vi "Example_Multiple.vi"() -> ()   [LabVIEW 2015, in "LXM32_Modbus_Serial.lvlib"]
uses:
  LXM32_Modbus_Serial.lvlib
  register_param.ctl
  <vilib>/Utility/sysdir.llb/System Directory Type.ctl
  <vilib>/Utility/file.llb/Write Delimited Spreadsheet (string).vi
  <vilib>/Utility/file.llb/Write Delimited Spreadsheet (DBL).vi
panel:
  in  "Stop":bool
  in  "LXM32 Port":refnum<visa-resource-name>
  out "chart10":dbl(graph) caption="Waveform Chart"
  out "chart9":dbl(graph) caption="Waveform Chart"
  out "chart8":dbl(graph) caption="Waveform Chart"
  out "chart7":dbl(graph) caption="Waveform Chart"
  out "chart6":dbl(graph) caption="Waveform Chart"
  out "chart5":dbl(graph) caption="Waveform Chart"
  out "chart4":dbl(graph) caption="Waveform Chart"
  out "chart3":dbl(graph) caption="Waveform Chart"
  out "chart2":dbl(graph) caption="Waveform Chart"
  out "chart1":dbl(graph) caption="Waveform Chart"
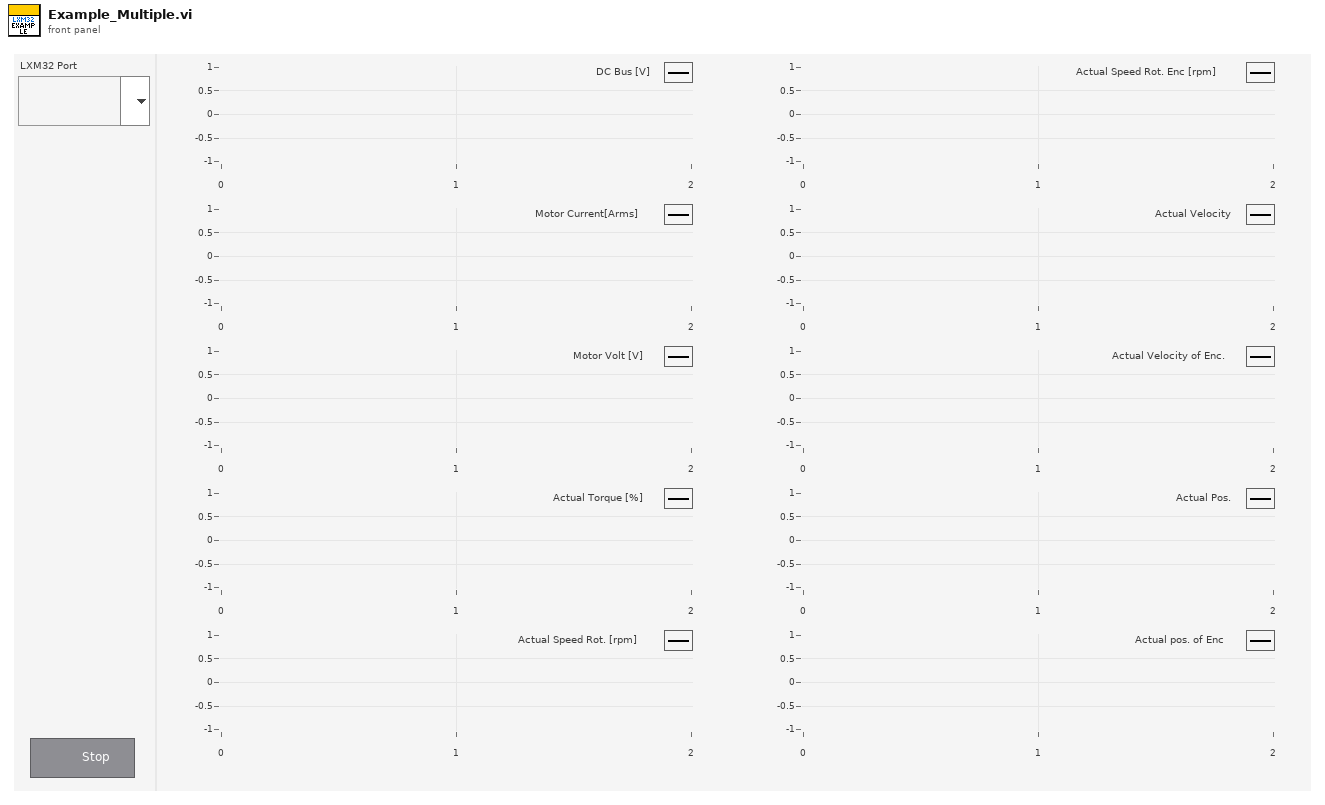
[diagram p1: front panel]
types:
  T1 = typedef "System Directory Type.ctl" = i32
  T2 = typedef "LXM32_Modbus_Serial.lvlib/register_param.ctl" = cluster{"name":string, "address":u16, "divisor":dbl}
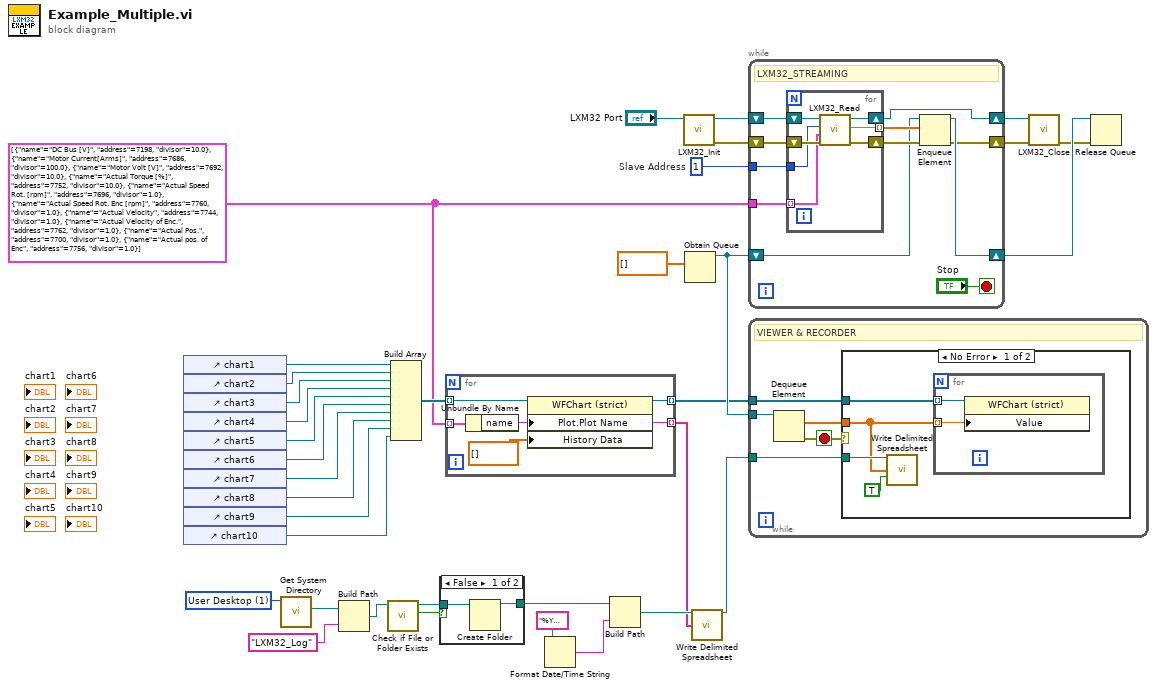
[diagram p0: block diagram]
diagram:
  w15 = T1 1 items=["User Home"=0, "User Desktop"=1, "User Documents"=2, "User Application Data"=3, "User Preferences"=4, "User Temporary"=5, "Public Documents"=6, "Public Application Data"=7, "Public Preferences"=8, "Public Cache"=13, "System Core Libraries"=9, "System Installed Libraries"=10, "Application Files"=11, "Boot Volume Root"=12] ("system directory type")
  w34 = u8 1  # Slave Address
  w1 = T2[] [{"name"="DC Bus [V]", "address"=7198, "divisor"=10.0}, {"name"="Motor Current[Arms]", "address"=7686, "divisor"=100.0}, {"name"="Motor Volt [V]", "address"=7692, "divisor"=10.0}, {"name"="Actual Torque [%]", "address"=7752, "divisor"=10.0}, {"name"="Actual Speed Rot. [rpm]", "address"=7696, "divisor"=1.0}, {"name"="Actual Speed Rot. Enc [rpm]", "address"=7760, "divisor"=1.0}, {"name"="Actual Velocity", "address"=7744, "divisor"=1.0}, {"name"="Actual Velocity of Enc.", "address"=7762, "divisor"=1.0}, {"name"="Actual Pos.", "address"=7700, "divisor"=1.0}, {"name"="Actual pos. of Enc", "address"=7756, "divisor"=1.0}]
  n1 = control-ref of="chart1"() -> (w27:refnum<vi>)
  n2 = control-ref of="chart2"() -> (w26:refnum<vi>)
  n3 = control-ref of="chart3"() -> (w25:refnum<vi>)
  n4 = control-ref of="chart4"() -> (w24:refnum<vi>)
  n5 = control-ref of="chart5"() -> (w23:refnum<vi>)
  n6 = control-ref of="chart6"() -> (w22:refnum<vi>)
  n7 = control-ref of="chart7"() -> (w21:refnum<vi>)
  n8 = control-ref of="chart8"() -> (w20:refnum<vi>)
  n9 = control-ref of="chart9"() -> (w19:refnum<vi>)
  n10 = control-ref of="chart10"() -> (w18:refnum<vi>)
  n11 = call <vilib>:"Get System Directory.vi"("system directory type"=w15) -> ("system directory"=w14:path)  [unwired: 10 in]
  n12 = Build Path(base path=w14, name or relative path="LXM32_Log") -> (appended path=w12:path)
  n13 = call <vilib>:"Check if File or Folder Exists.vi"("path"=w12) -> ("file or folder exists?"=w11:bool, "dup path"=w10:path)  [unwired: 8 in, 1 out]
  n14 = Build Array(w27, w26, w25, w24, w23, w22, w21, w20, w19, w18) -> (w17:refnum<vi>[])
  n15 = case shown="False" w11 {
    tunnel: w10 -> [w37 w38]
    tunnel: [w36 w38] -> w8
    frame False {
      n16 = Create Folder(path (use dialog)=w37) -> (created path=w36:path)  [unwired: 2 in, 2 out]
    }
    frame True {
    }
  }
  n17 = for {
    tunnel: w17 -> [w43] mode=indexing
    tunnel: w1 -> [w42] mode=indexing
    tunnel: [w40] -> w16 mode=indexing
    tunnel: [w39] -> w5 mode=indexing
    n18 = Unbundle By Name(w42) -> ("name"=w39:string)
    n19 = property class="WFChart (strict)"(reference=w43, "Plot.Plot Name"=w39, "History Data"=dbl[] []) -> (reference out=w40:refnum<vi>)  [unwired: 1 in, 1 out]
  }
  n20 = Format Date/Time String(time format string (%c)="%Y%m%d_%H%M%S.txt") -> (date/time string=w7:string)  [unwired: 2 in]
  n21 = Build Path(base path=w8, name or relative path=w7) -> (appended path=w6:path)
  n22 = call "LXM32_Init.vi"("VISA resource name"="LXM32 Port") -> ("error out"=w2:errorcluster, "VISA resource name out"=w3:refnum<visa-resource-name>)  [unwired: 9 in]
  n23 = Obtain Queue(element data type=dbl[] []) -> (queue out=w28:refnum<queue>)  [unwired: 4 in, 2 out]
  n24 = call-poly <vilib>:"Write Delimited Spreadsheet.vi"("file path (dialog if empty)"=w6, "1D data"=w5) -> ("new file path (Not A Path if cancelled)"=w4:path)  [unwired: 12 in, 1 out]
  n25 = while {
    shift-right: [w50] -> w33
    shift-left: w3 -> [w54]
    shift-right: [w45] -> w32
    shift-left: w2 -> [w53]
    tunnel: w1 -> [w52]
    tunnel: w34 -> [w51]
    shift-right: [w46] -> w30
    shift-left: w28 -> [w47]
    stop <- "Stop" stop-if-true
    # "LXM32_STREAMING"
    n26 = for {
      shift-right: [w59] -> w50
      shift-left: w54 -> [w61]
      shift-right: [w58] -> w49
      shift-left: w53 -> [w60]
      tunnel: w52 -> [w57] mode=indexing
      tunnel: w51 -> [w56]
      tunnel: [w55] -> w48 mode=indexing
      n27 = call "LXM32_Read.vi"("error in"=w60, "register param"=w57, "Slave Address"=w56, "VISA resource name"=w61) -> ("error out"=w58:errorcluster, "value"=w55:dbl, "VISA resource name out"=w59:refnum<visa-resource-name>)  [unwired: 5 in]
    }
    n28 = Enqueue Element(queue=w47, element=w48, error in (no error)=w49) -> (queue out=w46:refnum<queue>, error out=w45:errorcluster)  [unwired: 1 in, 1 out]
  }
  n29 = while {
    tunnel: w28 -> [w65]
    tunnel: w16 -> [w64]
    tunnel: w4 -> [w63]
    stop <- w66 stop-if-true
    # "VIEWER & RECORDER"
    n30 = Dequeue Element(queue=w65) -> (element=w62:dbl[], error out=w66:errorcluster)  [unwired: 2 in, 2 out]
    n31 = case shown="No Error" w66 {
      tunnel: w64 -> [w70 _]
      tunnel: w63 -> [w69 _]
      tunnel: w62 -> [w68 _]
      frame No Error {
        n32 = call-poly <vilib>:"Write Delimited Spreadsheet.vi"("file path (dialog if empty)"=w69, "1D data"=w68, "append to file? (F)"=TRUE) -> ()  [unwired: 11 in, 2 out]
        n33 = for {
          tunnel: w68 -> [w72] mode=indexing
          tunnel: w70 -> [w71] mode=indexing
          n34 = property class="WFChart (strict)"(reference=w71, "Value"=w72) -> ()  [unwired: 1 in, 2 out]
        }
      }
      frame Error {
      }
    }
  }
  n35 = call "LXM32_Close.vi"("error in"=w32, "VISA resource name"=w33) -> ("error out"=w29:errorcluster)  [unwired: 9 in]
  n36 = Release Queue(queue=w30, error in (no error)=w29) -> ()  [unwired: 1 in, 3 out]
